vi "test CAN Cyclic Loopback.vi"(8 "error in (no error)":errorcluster, 11 "TestCase in":refnum<class "CAN Loopback Tests.lvclass">) -> (0 "error out":errorcluster, 3 "TestCase out":refnum<class "CAN Loopback Tests.lvclass">)   [LabVIEW 2017, in "CAN Loopback Tests.lvclass"]
uses:
  CAN Loopback Tests.lvclass
  C:/Users/nitest/Documents/ni-official/niveristand-custom-device-testing-tools/VeriStandTestCase/VeriStandTestCase.lvclass
  70f1795c-6642-4f2f-bc4d-5f93b5bfa402.vi
  <vilib>/NI Veristand/Execution/Workspace/NI VeriStand - Set Multiple Channel Values.vi
  <vilib>/NI Veristand/Execution/Workspace/NI VeriStand - Get Multiple Channel Values.vi
  <vilib>/addons/_JKI Toolkits/VI Tester/TestCase.llb/TestCase.lvclass
  <vilib>/NI VeriStand/Execution/Workspace/NI_VS Workspace ExecutionAPI.lvlib
  C:/Program Files (x86)/National Instruments/LabVIEW 2017/vi.lib/addons/_JKI Toolkits/VI Tester/TestCase.llb/TestCase.lvclass
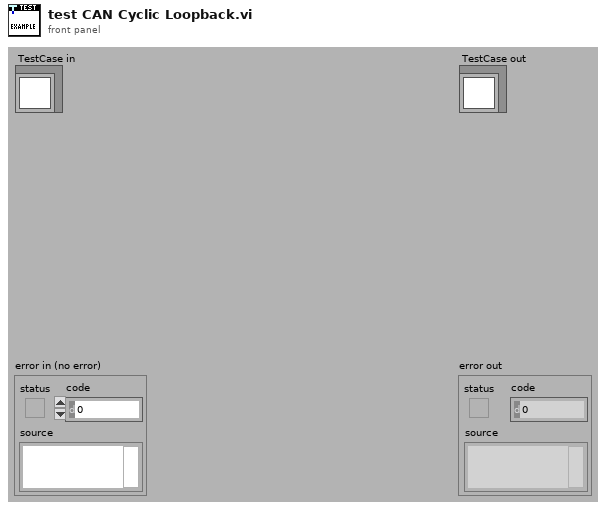
[diagram p1: front panel]
types:
  T1 = typedef "NI_VS Workspace ExecutionAPI.lvlib/WorkspaceAPI.ctl" = refnum<k24>
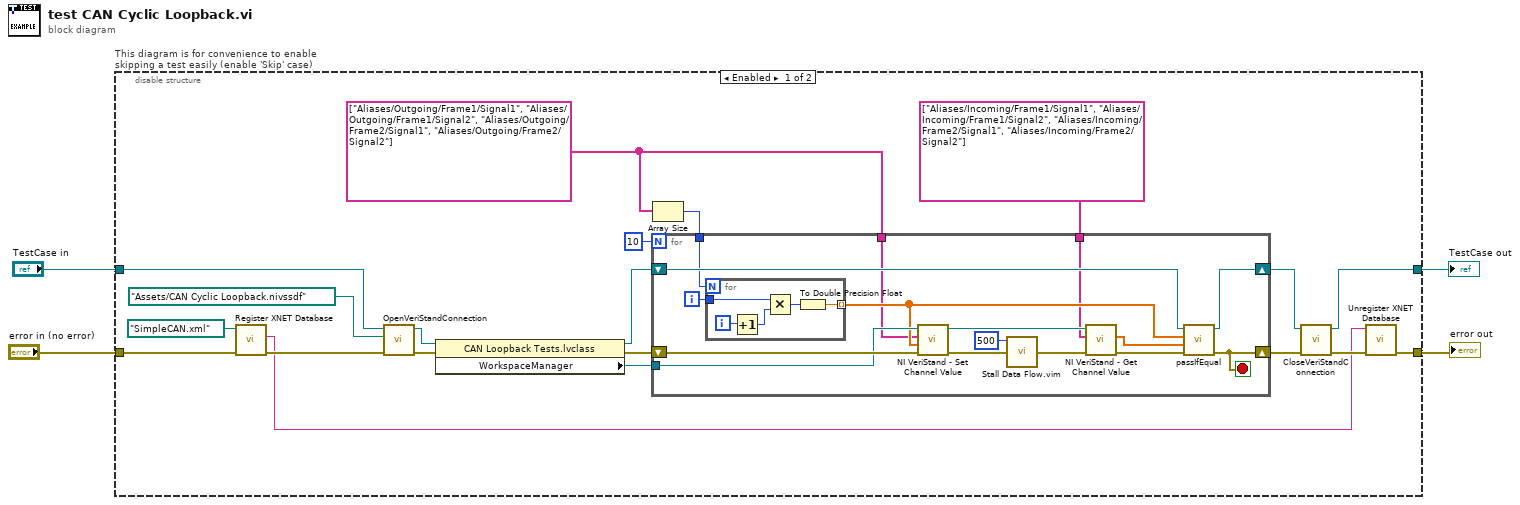
[diagram p0: block diagram]
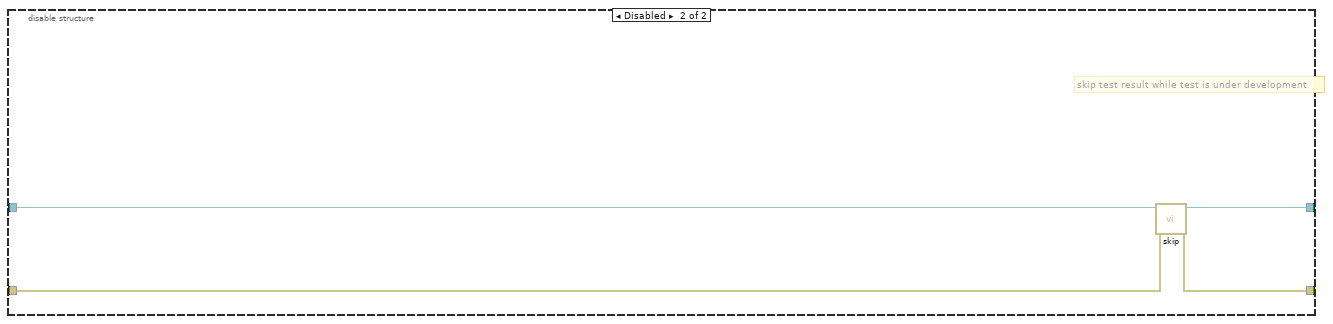
[diagram p2: hidden frame]
diagram:
  n1 = disable-structure "This diagram is for convenience to enable skipping a test easily (enable 'Skip' case)" shown="Enabled" {
    disable-tunnel: "TestCase in" -> [w24 w49]
    disable-tunnel: [w17 w47] -> w1
    disable-tunnel: [w7 w48] -> w3
    disable-tunnel: "error in (no error)" -> [w9 w46]
    frame Enabled {
      w13 = string[] ["Aliases/Outgoing/Frame1/Signal1", "Aliases/Outgoing/Frame1/Signal2", "Aliases/Outgoing/Frame2/Signal1", "Aliases/Outgoing/Frame2/Signal2"]
      n2 = call "Register XNET Database.vi"("error in (no error)"=w9, "database path"=path "SimpleCAN.xml") -> ("error out"=w8:errorcluster, "alias"=w5:string)  [unwired: 8 in]
      n3 = call-dynamic "OpenVeriStandConnection.vi"("error in (no error)"=w8, "System Definition File"=path "Assets/CAN Cyclic Loopback.nivssdf", "VeriStand Test Case in"=w24) -> ("error out"=w21:errorcluster, "VeriStand Test Case out"=w22:refnum<class "CAN Loopback Tests.lvclass">)  [unwired: 6 in, 1 out]
      n4 = property class="CAN Loopback Tests.lvclass"(reference=w22, error in=w21) -> (reference out=w18:refnum<class "CAN Loopback Tests.lvclass">, error out=w20:errorcluster, "WorkspaceManager"=w19:T1)
      n5 = Array Size(array=w13) -> (size(s)=w12:i32)
      n6 = for {
        N: 10 -> [_]
        shift-right: [w25] -> w15
        shift-left: w20 -> [w40]
        shift-right: [w32] -> w16
        shift-left: w18 -> [w31]
        tunnel: w19 -> [w39]
        tunnel: string[] ["Aliases/Incoming/Frame1/Signal1", "Aliases/Incoming/Frame1/Signal2", "Aliases/Incoming/Frame2/Signal1", "Aliases/Incoming/Frame2/Signal2"] -> [w28]
        tunnel: w13 -> [w27]
        tunnel: w12 -> [w26]
        i -> [w38]
        stop <- w25 stop-if-true
        n7 = for {
          N: w26 -> [_]
          tunnel: [w45] -> w29 mode=indexing
          tunnel: w38 -> [w44]
          i -> [w43]
          n8 = Increment(x=w43) -> (x+1=w42:i32)
          n9 = Multiply(x=w44, y=w42) -> (x*y=w41:i32)
          n10 = To Double Precision Float(number=w41) -> (double precision float=w45:dbl)
        }
        n11 = call-poly <vilib>:"NI VeriStand - Set Channel Value.vi"("error in (no error)"=w40, "Values"=w29, "Channels"=w27, "WorkspaceManager in"=w39) -> ("error out"=w37:errorcluster, "WorkspaceManager out"=w33:T1)  [unwired: 6 in]
        n12 = call "Stall Data Flow.vim"("value in"=w37, "milliseconds to wait"=u32 500) -> ("value out"=w36:errorcluster)  [unwired: 1 out]
        n13 = call-poly <vilib>:"NI VeriStand - Get Channel Value.vi"("error in (no error)"=w36, "Channels"=w28, "WorkspaceManager in"=w33) -> ("error out"=w35:errorcluster, "Values"=w30:dbl[])  [unwired: 6 in, 1 out]
        n14 = call-dynamic "passIfEqual.vi"("error in (no error)"=w35, "y"=w30, "x"=w29, "TestCase in"=w31) -> ("error out"=w25:errorcluster, "TestCase out"=w32:refnum<class "CAN Loopback Tests.lvclass">)  [unwired: 6 in]
      }
      n15 = call-dynamic "CloseVeriStandConnection.vi"("error in (no error)"=w15, "VeriStand Test Case in"=w16) -> ("error out"=w6:errorcluster, "VeriStand Test Case out"=w17:refnum<class "CAN Loopback Tests.lvclass">)  [unwired: 8 in]
      n16 = call "Unregister XNET Database.vi"("error in (no error)"=w6, "alias"=w5) -> ("error out"=w7:errorcluster)  [unwired: 9 in]
    }
    frame Disabled {
      # "skip test result while test is under development"
      n17 = call <vilib>:"skip.vi"("error in (no error)"=w46, "TestCase in"=w49) -> ("error out"=w48:errorcluster, "TestCase out"=w47:refnum<class "CAN Loopback Tests.lvclass">)  [unwired: 8 in]
    }
  }
  "error out" <- w3
  "TestCase out" <- w1
